vi "Reset Min and Max.vi"(8 "error in (no error)":errorcluster, 10 "Reset Min/Max Data (T: Yes)":bool=TRUE, 11 "VISA resource name":refnum<visa-resource-name>) -> (0 "error out":errorcluster, 3 "VISA resource name out":refnum<visa-resource-name>)   [LabVIEW 2012, in "Lake Shore 335.lvlib"]
doc: "Resets the Min/Max data function. Minimum and maximum data for both inputs is reset."
uses:
  <instrlib>/lake shore 335/Temperature control panel Folder/C/Program Files/National Instruments/LabVIEW 2013/instr.lib/lake shore 335/Lake Shore 335.lvlib
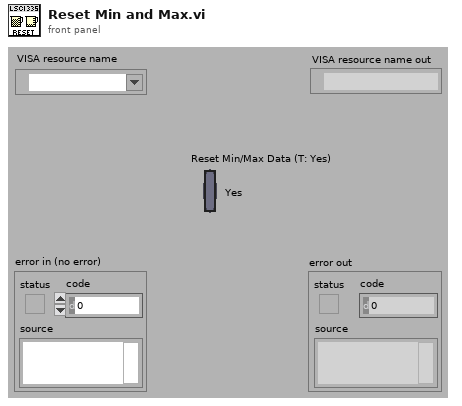
[diagram p1: front panel]
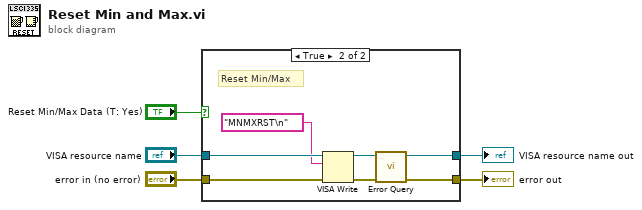
[diagram p0: block diagram]
diagram:
  n1 = case shown="True" "Reset Min/Max Data (T: Yes)" {
    tunnel: "VISA resource name" -> [w7 w14]
    tunnel: "error in (no error)" -> [w6 w13]
    tunnel: [w7 w10] -> w3
    tunnel: [w6 w9] -> w2
    frame False {
      # "Do not reset Min/Max"
    }
    frame True {
      # "Reset Min/Max"
      n2 = VISA Write(VISA resource name=w14, write buffer="MNMXRST\n", error in (no error)=w13) -> (VISA resource name out=w11:refnum<visa-resource-name>, error out=w12:errorcluster)  [unwired: 1 out]
      n3 = call <instrlib>:"Error Query.vi"("error in (no error)"=w12, "VISA resource name"=w11) -> ("error out"=w9:errorcluster, "VISA resource name out"=w10:refnum<visa-resource-name>)  [unwired: 7 in, 1 out]
    }
  }
  "VISA resource name out" <- w3
  "error out" <- w2
